vi "ArrayToString.vi"(0 "Header":string, 1 "Format":string, 2 "Input 1D array":dbl[](array[numeric]), 3 "Unit":string) -> (7 "Output 1D array":string[](array[string]))   [LabVIEW 2016]
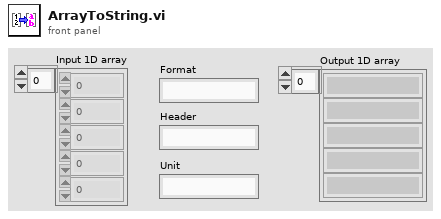
[diagram p1: front panel]
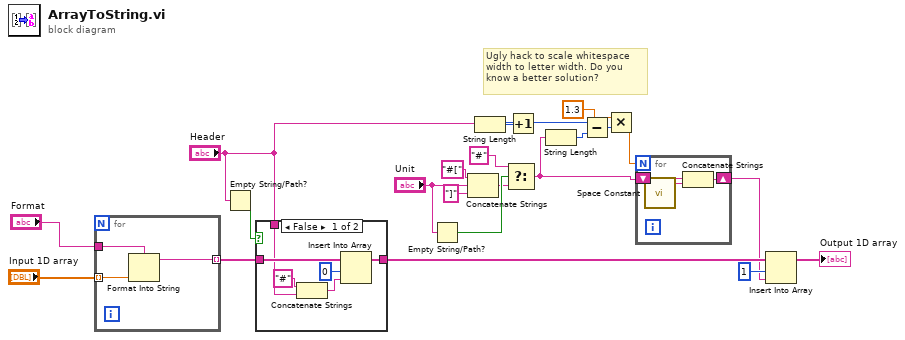
[diagram p0: block diagram]
diagram:
  # "Ugly hack to scale whitespace \nwidth to letter width. Do you\nknow a better solution?"
  n1 = for {
    tunnel: "Input 1D array" -> [w25] mode=indexing
    tunnel: "Format" -> [w24]
    tunnel: [w23] -> w20 mode=indexing
    n2 = Format Into String(format string=w24, w25) -> (resulting string=w23:string)  [unwired: 2 in, 1 out]
  }
  n3 = Empty String/Path?(string/path="Header") -> (empty?=w19:bool)
  n4 = case shown="False" w19 {
    tunnel: w20 -> [w31 w32]
    tunnel: "Header" -> [w27 _]
    tunnel: [w29 w32] -> w18
    frame False {
      n5 = Concatenate Strings("#" ("string"), w27) -> (w26:string)
      n6 = Insert Into Array(array=w31, index=0, new element=w26) -> (w29:string[])
    }
    frame True {
    }
  }
  n7 = Empty String/Path?(string/path="Unit") -> (empty?=w12:bool)
  n8 = Concatenate Strings("#[" ("string"), "Unit", "]" ("string")) -> (w10:string)
  n9 = String Length(string="Header") -> (length=w8:i32)
  n10 = Select(t="#" ("string"), s=w12, f=w10) -> (s? t:f=w3:string)
  n11 = Increment(x=w8) -> (x+1=w6:i32)
  n12 = String Length(string=w3) -> (length=w7:i32)
  n13 = Subtract(x=w6, y=w7) -> (x-y=w5:i32)
  n14 = Multiply(x=1.3, y=w5) -> (x*y=w2:dbl)
  n15 = for {
    N: w2 -> [_]
    shift-right: [w35] -> w4
    shift-left: w3 -> [w33]
    n16 = call <vilib>:"Space Constant.vi"() -> ("String"=w34:string)
    n17 = Concatenate Strings(w33, w34) -> (w35:string)
  }
  n18 = Insert Into Array(array=w18, index=1, new element=w4) -> (→"Output 1D array":string[])
